vi "Schmitt_Trigger.vi"(2 "lo":dbl(knob) scale=0.0..10.0, 3 "in":dbl(knob) scale=0.0..10.0, 4 "hi":dbl(knob) scale=0.0..10.0) -> (0 "inv out":bool, 1 "out":bool)   [LabVIEW 2015]
doc: "Help by FRC Team 836 - The RoboBees\n\nSchmitt Trigger\n\nVI Description: This is a code implementation of the electronic circuit behavior invented by Otto Schmitt in 1938. It provides a logical True OUT when the input IN exceeds the value for HI, but does not then return a logical False until IN falls below the value for LO. Because of this behavior, it acts as a threshold detector with hysterisis (which just means it acts differently depending on which direction the input is changing). It can be used to threshold an Analog input, insensitive to noise, as long as the noise level isn't too great.\n\nInputs:\nIN - The numeric signal being tested for threshold.\nHI - The high threshold value, above which will result in a True OUT.\nLO -The low threshold value, below which will result in a False OUT.\n\nOutputs:\nOUT - Result of appliying IN to threshold test.\nINV OUT - Inverse of OUT, representing an Inverting Schmitt-Trigger.\n\nImplementation:\nDetermine values for HI and LO to create a seperation larger than the random variation (noise) present in IN.\n\nExecution Properties:\nDebugging is disabled for performance improvement.\nReentrancy is set to Preallocated Clone, which allows the VI to be used in multiple places, without confusing indivual VI's State.\n\nAttribution: This code was provided by Altenbach on a NI LabVIEW Forum post in 2005\nhttp://forums.ni.com/t5/LabVIEW/Schmitt-Trigger/td-p/300823\nwith minor modification to include an output for an Inverting Schmitt-Trigger\n\nFIRST Team 836, RoboBees ... Cross the threshold to a career in STEM and create your own inventions!"
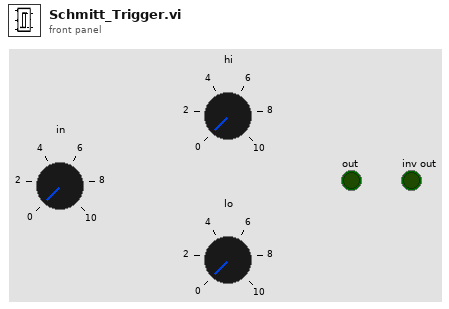
[diagram p1: front panel]
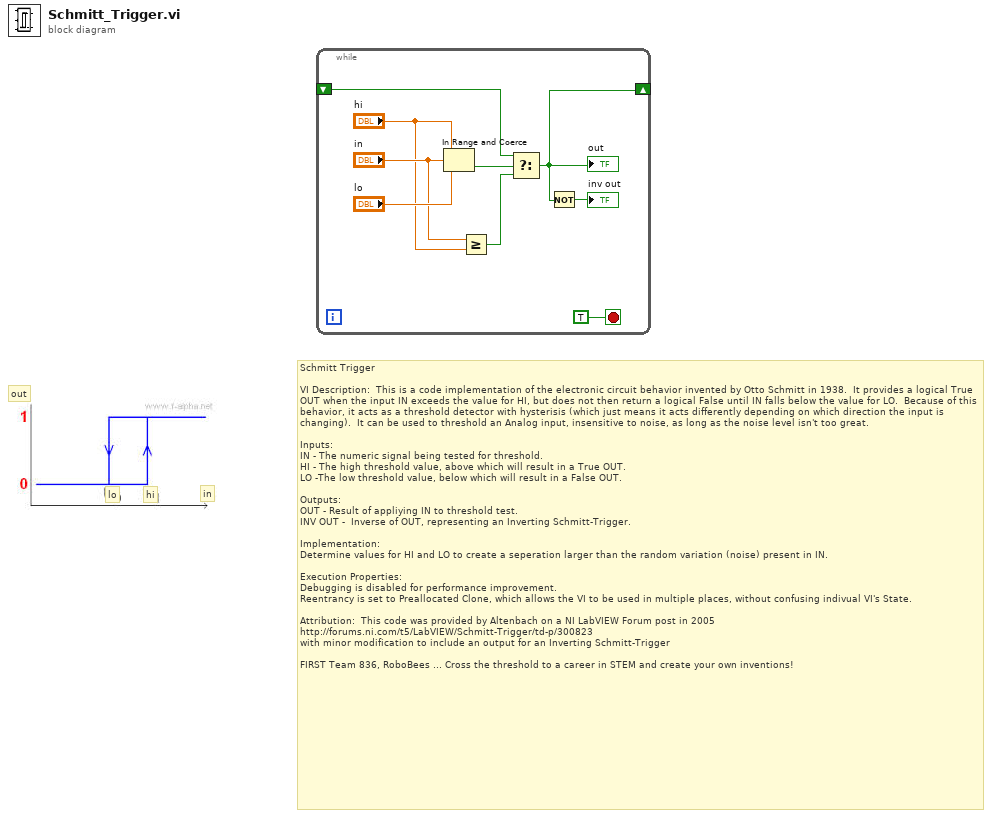
[diagram p0: block diagram]
diagram:
  # "out"
  # "in"
  # "lo"
  # "hi"
  # "Schmitt Trigger\n\nVI Description:  This is a code implementation of the electronic circuit behavior invented by Otto Schmitt in 1938.  It provides a logical True OUT when the input IN exceeds the value for HI, but does not then return a logical False until IN falls below the value for LO.  Because of this behavior, it acts as a threshold detector with hysterisis (which just means it acts differently depending on which direction the input is changing).  It can be used to threshold an Analog input, insensitive to noise, as long as the noise level isn't too great.\n\nInputs:\nIN - The numeric signal being tested for threshold.\nHI - The high threshold value, above which will result in a True OUT.\nLO -The low threshold value, below which will result in a False OUT.\n\nOutputs:\nOUT - Result of appliying IN to threshold test.\nINV OUT -  Inverse of OUT, representing an Inverting Schmitt-Trigger.\n\nImplementation:\nDetermine values for HI and LO to create a seperation larger than the random variation (noise) present in IN.\n\nExecution Properties:\nDebugging is disabled for performance improvement.\nReentrancy is set to Preallocated Clone, which allows the VI to be used in multiple places, without confusing indivual VI's State.\n\nAttribution:  This code was provided by Altenbach on a NI LabVIEW Forum post in 2005\nhttp://forums.ni.com/t5/LabVIEW/Schmitt-Trigger/td-p/300823\nwith minor modification to include an output for an Inverting Schmitt-Trigger\n\nFIRST Team 836, RoboBees ... Cross the threshold to a career in STEM and create your own inventions!"
  n1 = while {
    shift-right: [w2] -> _
    shift-left: _ -> [w3]
    stop <- TRUE stop-if-true
    n2 = In Range and Coerce(upper limit="hi", x="in", lower limit="lo") -> (In Range?=w7:bool)  [unwired: 1 out]
    n3 = Greater Or Equal?(x="in", y="hi") -> (x >= y?=w4:bool)
    n4 = Select(t=w3, s=w7, f=w4) -> (s? t:f=w2:bool)
    "out" <- w2
    n5 = Not(x=w2) -> (.not. x?=→"inv out":bool)
  }
